vi "Fire Stop Helper Loop Event.vi"(11 "Acquisition UI in":refnum<class "Acquisition UI.lvclass">) -> (3 "Acquisition UI out":refnum<class "Acquisition UI.lvclass">)   [LabVIEW 2018, in "Acquisition UI.lvlib" / "Acquisition UI.lvclass"]
uses:
  Acquisition UI.lvclass
  Acquisition UI.lvclass/Acquisition UI.ctl
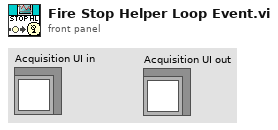
[diagram p1: front panel]
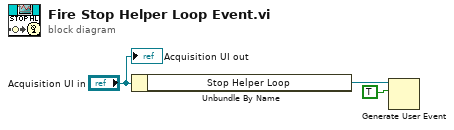
[diagram p0: block diagram]
diagram:
  n1 = Unbundle By Name("Acquisition UI in") -> ("Stop Helper Loop"=w3:refnum<user-event>)
  n2 = Generate User Event(user event=w3, event data cluster=TRUE ("event data")) -> ()  [unwired: 2 in, 2 out]
  "Acquisition UI out" <- "Acquisition UI in"
